vi "Arm Position Corection.vi"(10 "Potentiometer Value":dbl) -> (2 "Arm Position":dbl)   [LabVIEW 2013]
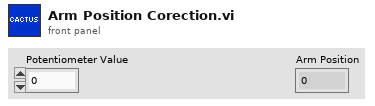
[diagram p1: front panel]
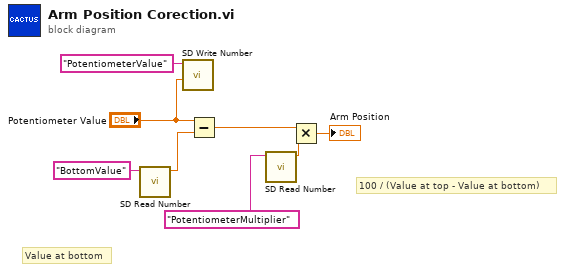
[diagram p0: block diagram]
diagram:
  # "100 / (Value at top - Value at bottom)"
  # "Value at bottom"
  n1 = call <vilib>:"SD Read Number.vi"("Name"="BottomValue") -> ("Numeric"=w6:dbl)  [unwired: 8 in, 2 out]
  n2 = call <vilib>:"SD Write Number.vi"("Numeric"="Potentiometer Value", "Name"="PotentiometerValue") -> ()  [unwired: 8 in, 2 out]
  n3 = Subtract(x="Potentiometer Value", y=w6) -> (x-y=w8:dbl)
  n4 = call <vilib>:"SD Read Number.vi"("Name"="PotentiometerMultiplier") -> ("Numeric"=w2:dbl)  [unwired: 8 in, 2 out]
  n5 = Multiply(x=w8, y=w2) -> (x*y=→"Arm Position":dbl)
